vi "Register gRPC Messages.vi"(8 "error in (no error)":errorcluster, 11 "gRPC ID":T1) -> (0 "error out":errorcluster, 3 "gRPC ID Out":T1)   [LabVIEW 2021, in "CIF_Plugin_Core_client.lvlib"]
uses:
  CIF_Plugin_Core_client.lvlib
  <vilib>/gRPC/LabVIEW gRPC Library/Shared/grpcId.ctl
  <vilib>/gRPC/LabVIEW gRPC Library/Server API/typeDefs/Message Metadata.ctl
  <vilib>/gRPC/LabVIEW gRPC Library/Server API/typeDefs/Message Element Metadata.ctl
  <vilib>/gRPC/LabVIEW gRPC Library/Server API/typeDefs/Message Element Type.ctl
  <vilib>/gRPC/LabVIEW gRPC Library/Server API/typeDefs/Enum Metadata.ctl
  <vilib>/gRPC/LabVIEW gRPC Library/grpc-lvsupport-release.lvlib
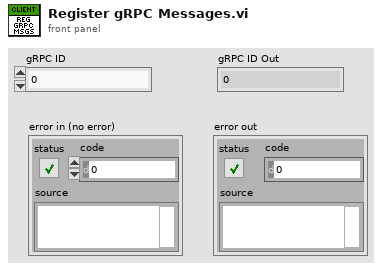
[diagram p1: front panel]
types:
  T1 = typedef "grpc-lvsupport-release.lvlib/grpcId.ctl" = u64
  T2 = typedef "grpc-lvsupport-release.lvlib/Enum Metadata.ctl" = cluster{"Version":i32, "Name":string, "Type Url":string, "Enum Values":string, "Allow Alias":bool}
  T3 = typedef "grpc-lvsupport-release.lvlib/Message Metadata.ctl" = cluster{"Version":i32, "Name":string, "Type Url":string, "Elements":T4[], "Has Oneof":bool}
  T4 = typedef "grpc-lvsupport-release.lvlib/Message Element Metadata.ctl" = cluster{"Field Name":string, "Embedded Message Name":string, "Protobuf Index":i32, "MessageElementType":T5, "Repeated":bool, "Is in Oneof":bool, "Oneof Container Name":string}
  T5 = typedef "grpc-lvsupport-release.lvlib/Message Element Type.ctl" = enum32{"Int32Value", "FloatValue", "DoubleValue", "BoolValue", "StringValue", "MessageValue", "Int64Value", "UInt32Value", "UInt64Value", "EnumValue", "Bytes", "Fixed64", "Fixed32", "SFixed64", "SFixed32", "SInt64", "SInt32"}
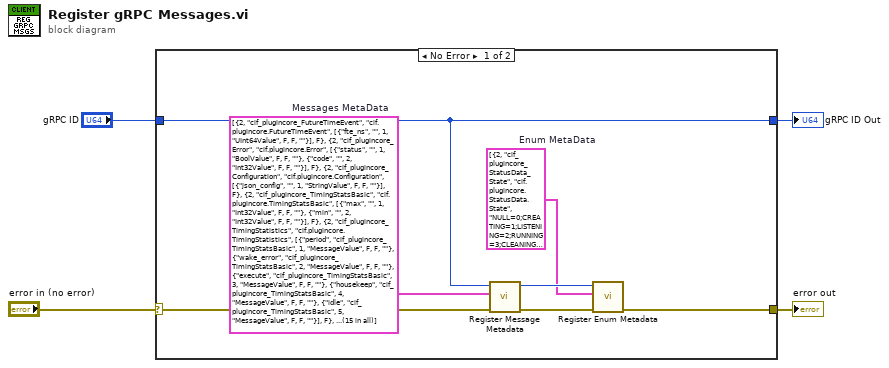
[diagram p0: block diagram]
diagram:
  n1 = case shown="No Error" "error in (no error)" {
    selector: "error in (no error)" -> [w10 w13]
    tunnel: [w9 w12] -> w1
    tunnel: [w6 w13] -> w4
    tunnel: "gRPC ID" -> [w9 w12]
    frame No Error {
      w5 = T2[] [{"Version"=2, "Name"="cif_plugincore_StatusData_State", "Type Url"="cif.plugincore.StatusData.State", "Enum Values"="NULL=0;CREATING=1;LISTENING=2;RUNNING=3;CLEANINGUP=4;DESTROYING=5", "Allow Alias"=FALSE}]  # Enum MetaData
      w11 = T3[] [{"Version"=2, "Name"="cif_plugincore_FutureTimeEvent", "Type Url"="cif.plugincore.FutureTimeEvent", "Elements"=[{"Field Name"="fte_ns", "Embedded Message Name"="", "Protobuf Index"=1, "MessageElementType"=enum."UInt64Value", "Repeated"=FALSE, "Is in Oneof"=FALSE, "Oneof Container Name"=""}], "Has Oneof"=FALSE}, {"Version"=2, "Name"="cif_plugincore_Error", "Type Url"="cif.plugincore.Error", "Elements"=[{"Field Name"="status", "Embedded Message Name"="", "Protobuf Index"=1, "MessageElementType"=enum."BoolValue", "Repeated"=FALSE, "Is in Oneof"=FALSE, "Oneof Container Name"=""}, {"Field Name"="code", "Embedded Message Name"="", "Protobuf Index"=2, "MessageElementType"=enum."Int32Value", "Repeated"=FALSE, "Is in Oneof"=FALSE, "Oneof Container Name"=""}], "Has Oneof"=FALSE}, {"Version"=2, "Name"="cif_plugincore_Configuration", "Type Url"="cif.plugincore.Configuration", "Elements"=[{"Field Name"="json_config", "Embedded Message Name"="", "Protobuf Index"=1, "MessageElementType"=enum."StringValue", "Repeated"=FALSE, "Is in Oneof"=FALSE, "Oneof Container Name"=""}], "Has Oneof"=FALSE}, {"Version"=2, "Name"="cif_plugincore_TimingStatsBasic", "Type Url"="cif.plugincore.TimingStatsBasic", "Elements"=[{"Field Name"="max", "Embedded Message Name"="", "Protobuf Index"=1, "MessageElementType"=enum."Int32Value", "Repeated"=FALSE, "Is in Oneof"=FALSE, "Oneof Container Name"=""}, {"Field Name"="min", "Embedded Message Name"="", "Protobuf Index"=2, "MessageElementType"=enum."Int32Value", "Repeated"=FALSE, "Is in Oneof"=FALSE, "Oneof Container Name"=""}], "Has Oneof"=FALSE}, {"Version"=2, "Name"="cif_plugincore_TimingStatistics", "Type Url"="cif.plugincore.TimingStatistics", "Elements"=[{"Field Name"="period", "Embedded Message Name"="cif_plugincore_TimingStatsBasic", "Protobuf Index"=1, "MessageElementType"=enum."MessageValue", "Repeated"=FALSE, "Is in Oneof"=FALSE, "Oneof Container Name"=""}, {"Field Name"="wake_error", "Embedded Message Name"="cif_plugincore_TimingStatsBasic", "Protobuf Index"=2, "MessageElementType"=enum."MessageValue", "Repeated"=FALSE, "Is in Oneof"=FALSE, "Oneof Container Name"=""}, {"Field Name"="execute", "Embedded Message Name"="cif_plugincore_TimingStatsBasic", "Protobuf Index"=3, "MessageElementType"=enum."MessageValue", "Repeated"=FALSE, "Is in Oneof"=FALSE, "Oneof Container Name"=""}, {"Field Name"="housekeep", "Embedded Message Name"="cif_plugincore_TimingStatsBasic", "Protobuf Index"=4, "MessageElementType"=enum."MessageValue", "Repeated"=FALSE, "Is in Oneof"=FALSE, "Oneof Container Name"=""}, {"Field Name"="idle", "Embedded Message Name"="cif_plugincore_TimingStatsBasic", "Protobuf Index"=5, "MessageElementType"=enum."MessageValue", "Repeated"=FALSE, "Is in Oneof"=FALSE, "Oneof Container Name"=""}], "Has Oneof"=FALSE}, {"Version"=2, "Name"="cif_plugincore_FifoStatistics", "Type Url"="cif.plugincore.FifoStatistics", "Elements"=[{"Field Name"="from_t0", "Embedded Message Name"="cif_plugincore_TimingStatsBasic", "Protobuf Index"=1, "MessageElementType"=enum."MessageValue", "Repeated"=FALSE, "Is in Oneof"=FALSE, "Oneof Container Name"=""}, {"Field Name"="from_previous_plugin", "Embedded Message Name"="cif_plugincore_TimingStatsBasic", "Protobuf Index"=2, "MessageElementType"=enum."MessageValue", "Repeated"=FALSE, "Is in Oneof"=FALSE, "Oneof Container Name"=""}, {"Field Name"="output_error", "Embedded Message Name"="cif_plugincore_TimingStatsBasic", "Protobuf Index"=3, "MessageElementType"=enum."MessageValue", "Repeated"=FALSE, "Is in Oneof"=FALSE, "Oneof Container Name"=""}], "Has Oneof"=FALSE}, {"Version"=2, "Name"="cif_plugincore_MonitorDoubles", "Type Url"="cif.plugincore.MonitorDoubles", "Elements"=[{"Field Name"="double_1", "Embedded Message Name"="", "Protobuf Index"=1, "MessageElementType"=enum."DoubleValue", "Repeated"=FALSE, "Is in Oneof"=FALSE, "Oneof Container Name"=""}, {"Field Name"="double_2", "Embedded Message Name"="", "Protobuf Index"=2, "MessageElementType"=enum."DoubleValue", "Repeated"=FALSE, "Is in Oneof"=FALSE, "Oneof Container Name"=""}, {"Field Name"="double_3", "Embedded Message Name"="", "Protobuf Index"=3, "MessageElementType"=enum."DoubleValue", "Repeated"=FALSE, "Is in Oneof"=FALSE, "Oneof Container Name"=""}, {"Field Name"="double_4", "Embedded Message Name"="", "Protobuf Index"=4, "MessageElementType"=enum."DoubleValue", "Repeated"=FALSE, "Is in Oneof"=FALSE, "Oneof Container Name"=""}], "Has Oneof"=FALSE}, {"Version"=2, "Name"="cif_plugincore_MonitorU64", "Type Url"="cif.plugincore.MonitorU64", "Elements"=[{"Field Name"="u64_1", "Embedded Message Name"="", "Protobuf Index"=1, "MessageElementType"=enum."UInt64Value", "Repeated"=FALSE, "Is in Oneof"=FALSE, "Oneof Container Name"=""}, {"Field Name"="u64_2", "Embedded Message Name"="", "Protobuf Index"=2, "MessageElementType"=enum."UInt64Value", "Repeated"=FALSE, "Is in Oneof"=FALSE, "Oneof Container Name"=""}, {"Field Name"="u64_3", "Embedded Message Name"="", "Protobuf Index"=3, "MessageElementType"=enum."UInt64Value", "Repeated"=FALSE, "Is in Oneof"=FALSE, "Oneof Container Name"=""}, {"Field Name"="u64_4", "Embedded Message Name"="", "Protobuf Index"=4, "MessageElementType"=enum."UInt64Value", "Repeated"=FALSE, "Is in Oneof"=FALSE, "Oneof Container Name"=""}], "Has Oneof"=FALSE}, {"Version"=2, "Name"="cif_plugincore_MonitorI64", "Type Url"="cif.plugincore.MonitorI64", "Elements"=[{"Field Name"="i64_1", "Embedded Message Name"="", "Protobuf Index"=1, "MessageElementType"=enum."Int64Value", "Repeated"=FALSE, "Is in Oneof"=FALSE, "Oneof Container Name"=""}, {"Field Name"="i64_2", "Embedded Message Name"="", "Protobuf Index"=2, "MessageElementType"=enum."Int64Value", "Repeated"=FALSE, "Is in Oneof"=FALSE, "Oneof Container Name"=""}, {"Field Name"="i64_3", "Embedded Message Name"="", "Protobuf Index"=3, "MessageElementType"=enum."Int64Value", "Repeated"=FALSE, "Is in Oneof"=FALSE, "Oneof Container Name"=""}, {"Field Name"="i64_4", "Embedded Message Name"="", "Protobuf Index"=4, "MessageElementType"=enum."Int64Value", "Repeated"=FALSE, "Is in Oneof"=FALSE, "Oneof Container Name"=""}], "Has Oneof"=FALSE}, {"Version"=2, "Name"="cif_plugincore_StatusData", "Type Url"="cif.plugincore.StatusData", "Elements"=[{"Field Name"="state", "Embedded Message Name"="cif_plugincore_StatusData_State", "Protobuf Index"=1, "MessageElementType"=enum."EnumValue", "Repeated"=FALSE, "Is in Oneof"=FALSE, "Oneof Container Name"=""}, {"Field Name"="timing_statistics", "Embedded Message Name"="cif_plugincore_TimingStatistics", "Protobuf Index"=2, "MessageElementType"=enum."MessageValue", "Repeated"=FALSE, "Is in Oneof"=FALSE, "Oneof Container Name"=""}, {"Field Name"="fifo_statistics", "Embedded Message Name"="cif_plugincore_FifoStatistics", "Protobuf Index"=3, "MessageElementType"=enum."MessageValue", "Repeated"=FALSE, "Is in Oneof"=FALSE, "Oneof Container Name"=""}, {"Field Name"="error", "Embedded Message Name"="cif_plugincore_Error", "Protobuf Index"=4, "MessageElementType"=enum."MessageValue", "Repeated"=FALSE, "Is in Oneof"=FALSE, "Oneof Container Name"=""}, {"Field Name"="monitor_doubles", "Embedded Message Name"="cif_plugincore_MonitorDoubles", "Protobuf Index"=5, "MessageElementType"=enum."MessageValue", "Repeated"=FALSE, "Is in Oneof"=FALSE, "Oneof Container Name"=""}, {"Field Name"="monitor_u64s", "Embedded Message Name"="cif_plugincore_MonitorU64", "Protobuf Index"=6, "MessageElementType"=enum."MessageValue", "Repeated"=FALSE, "Is in Oneof"=FALSE, "Oneof Container Name"=""}, {"Field Name"="monitor_i64s", "Embedded Message Name"="cif_plugincore_MonitorI64", "Protobuf Index"=7, "MessageElementType"=enum."MessageValue", "Repeated"=FALSE, "Is in Oneof"=FALSE, "Oneof Container Name"=""}], "Has Oneof"=FALSE}, {"Version"=2, "Name"="cif_plugincore_Version", "Type Url"="cif.plugincore.Version", "Elements"=[{"Field Name"="major", "Embedded Message Name"="", "Protobuf Index"=1, "MessageElementType"=enum."UInt32Value", "Repeated"=FALSE, "Is in Oneof"=FALSE, "Oneof Container Name"=""}, {"Field Name"="minor", "Embedded Message Name"="", "Protobuf Index"=2, "MessageElementType"=enum."UInt32Value", "Repeated"=FALSE, "Is in Oneof"=FALSE, "Oneof Container Name"=""}, {"Field Name"="fix", "Embedded Message Name"="", "Protobuf Index"=3, "MessageElementType"=enum."UInt32Value", "Repeated"=FALSE, "Is in Oneof"=FALSE, "Oneof Container Name"=""}, {"Field Name"="build", "Embedded Message Name"="", "Protobuf Index"=4, "MessageElementType"=enum."UInt32Value", "Repeated"=FALSE, "Is in Oneof"=FALSE, "Oneof Container Name"=""}], "Has Oneof"=FALSE}, {"Version"=2, "Name"="cif_plugincore_TimingOverrides", "Type Url"="cif.plugincore.TimingOverrides", "Elements"=[{"Field Name"="override_timing", "Embedded Message Name"="", "Protobuf Index"=1, "MessageElementType"=enum."BoolValue", "Repeated"=FALSE, "Is in Oneof"=FALSE, "Oneof Container Name"=""}, {"Field Name"="period", "Embedded Message Name"="", "Protobuf Index"=2, "MessageElementType"=enum."DoubleValue", "Repeated"=FALSE, "Is in Oneof"=FALSE, "Oneof Container Name"=""}], "Has Oneof"=FALSE}, {"Version"=2, "Name"="cif_plugincore_PluginOverrides", "Type Url"="cif.plugincore.PluginOverrides", "Elements"=[{"Field Name"="timing_overrides", "Embedded Message Name"="cif_plugincore_TimingOverrides", "Protobuf Index"=1, "MessageElementType"=enum."MessageValue", "Repeated"=FALSE, "Is in Oneof"=FALSE, "Oneof Container Name"=""}], "Has Oneof"=FALSE}, {"Version"=2, "Name"="cif_plugincore_Status", "Type Url"="cif.plugincore.Status", "Elements"=[{"Field Name"="code", "Embedded Message Name"="", "Protobuf Index"=1, "MessageElementType"=enum."Int32Value", "Repeated"=FALSE, "Is in Oneof"=FALSE, "Oneof Container Name"=""}, {"Field Name"="message", "Embedded Message Name"="", "Protobuf Index"=2, "MessageElementType"=enum."StringValue", "Repeated"=FALSE, "Is in Oneof"=FALSE, "Oneof Container Name"=""}], "Has Oneof"=FALSE}, {"Version"=2, "Name"="cif_plugincore_Empty", "Type Url"="cif.plugincore.Empty", "Elements"=[], "Has Oneof"=FALSE}]  # Messages MetaData
      n2 = call <vilib>:"Register Message Metadata.vi"("error in"=w10, "Messages"=w11, "gRPCid in"=w9) -> ("error out"=w7:errorcluster, "gRPCid out"=w8:T1)  [unwired: 7 in]
      n3 = call <vilib>:"Register Enum Metadata.vi"("error in"=w7, "Enum Metadata"=w5, "gRPCid in"=w8) -> ("error out"=w6:errorcluster)  [unwired: 7 in, 1 out]
    }
    frame Error {
    }
  }
  "error out" <- w4
  "gRPC ID Out" <- w1
